vi "Unloading_OPEN_DOOR_ON_LOADED_status_Check.vi"(7 "CYCLE DATA IN":T1, 8 "error in":errorcluster) -> (0 "error out":errorcluster, 2 "search valid ?":bool, 5 "CYCLE DATA OUT":T1)   [LabVIEW 2017]
uses:
  Controls/Unload_Cyc_Data.ctl
  <vilib>/Utility/file.llb/Read Delimited Spreadsheet (string).vi
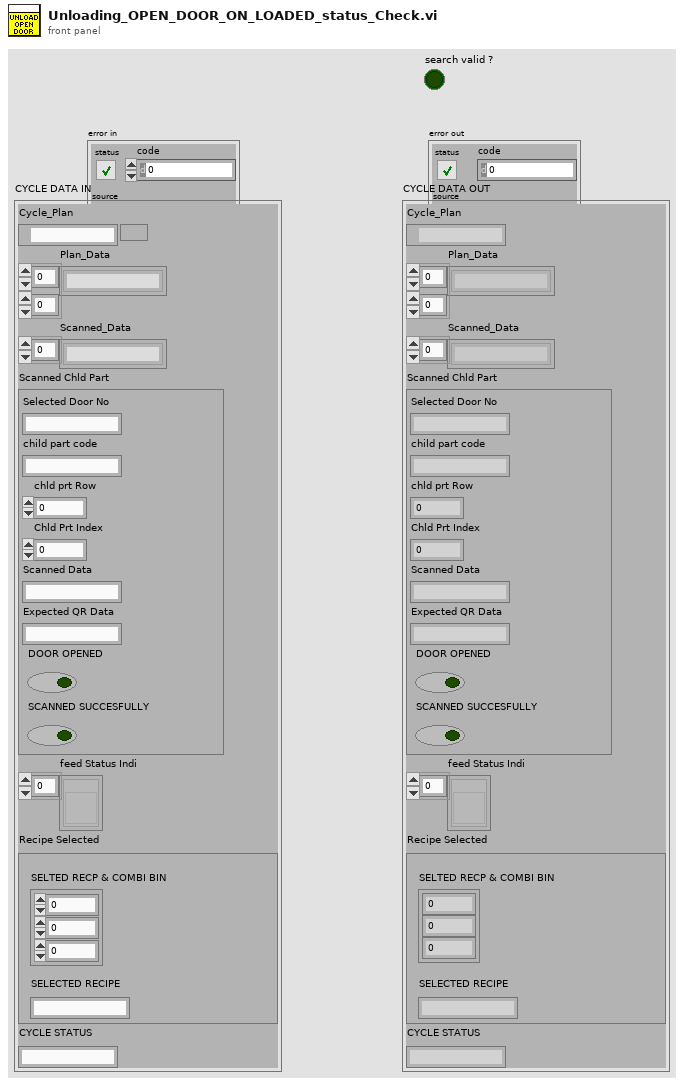
[diagram p1: front panel]
types:
  T1 = typedef "Unload_Cyc_Data.ctl" = cluster{"Cycle_Plan":path, "Plan_Data":string[][], "Scanned_Data":string[], "Scanned Chld Part":cluster{"Selected Door No":string, "child part code":string, "chld prt Row":i32, "Chld Prt Index":i32, "Scanned Data":string, "Expected QR Data":string, "DOOR OPENED":bool, "SCANNED SUCCESFULLY":bool}, "feed Status Indi":refnum<vi>[], "Recipe Selected":cluster{"SELTED RECP & COMBI BIN":cluster{"RECIPE INDEX":i32, "COMBI BIN":i32, "Section row no.":i32}, "SELECTED RECIPE":string}, "CYCLE STATUS":string}
  T2 = cluster{"RECIPE INDEX":i32, "COMBI BIN":i32, "Section row no.":i32}
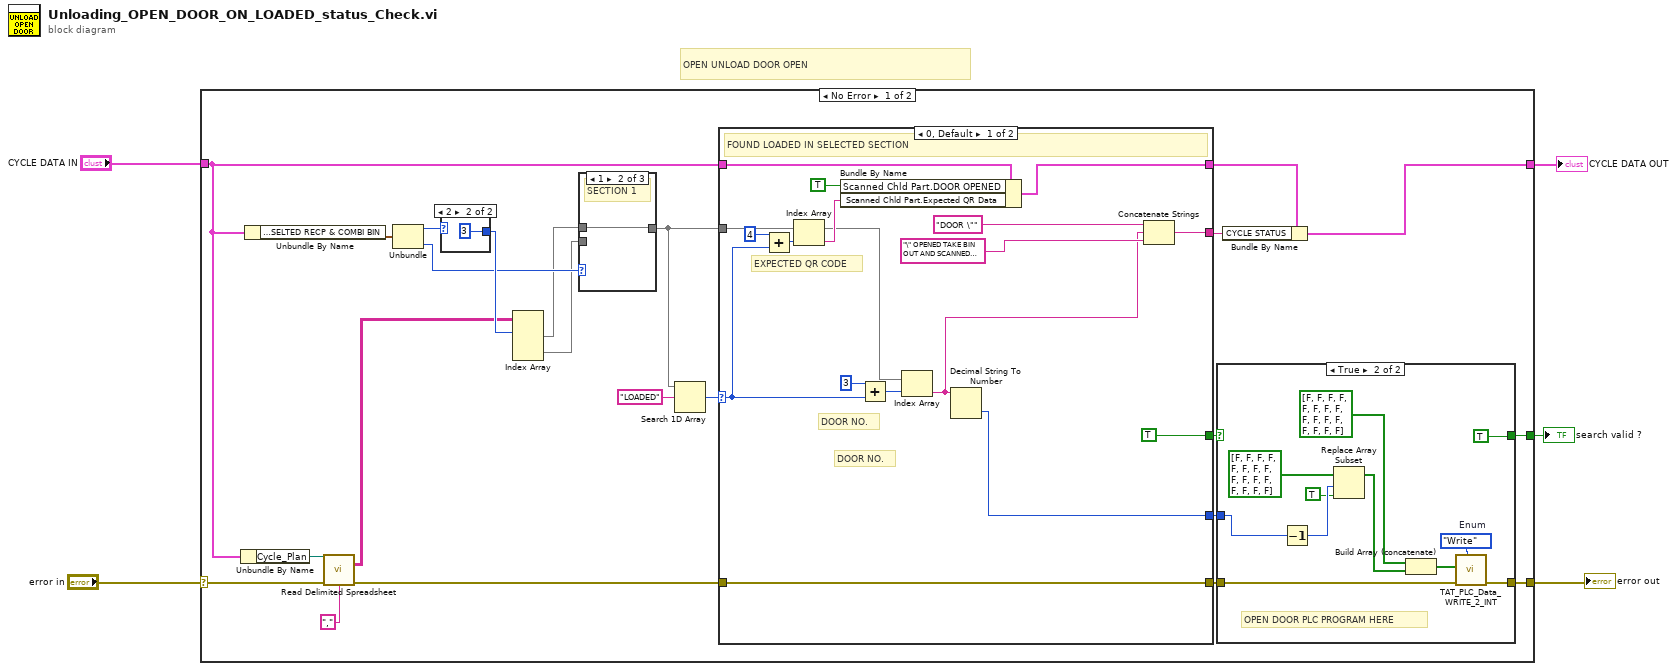
[diagram p0: block diagram]
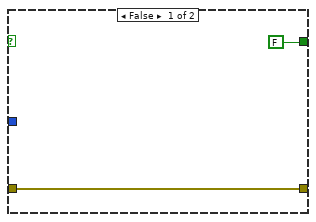
[diagram p2: hidden frame]
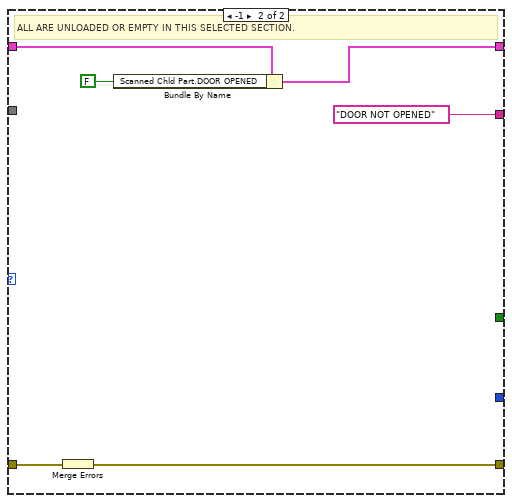
[diagram p3: hidden frame]
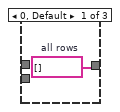
[diagram p4: hidden frame]
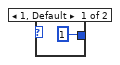
[diagram p6: hidden frame]
diagram:
  # "OPEN UNLOAD DOOR OPEN"
  n1 = case shown="No Error" "error in" {
    selector: "error in" -> [w25 w71]
    tunnel: [w18 w71] -> w4
    tunnel: [w13 w70] -> w2
    tunnel: "CYCLE DATA IN" -> [w21 w70]
    tunnel: [w15 _] -> w1
    frame No Error {
      n2 = Unbundle By Name(w21) -> ("Cycle_Plan"=w26:path)
      n3 = Unbundle By Name(w21) -> ("Recipe Selected.SELTED RECP & COMBI BIN"=w23:T2)
      n4 = call-poly <vilib>:"Read Delimited Spreadsheet.vi"("file path (dialog if empty)"=w26, "error in (no error)"=w25, "delimiter (\\t)"=",") -> ("all rows"=w19:string[][], "error out"=w24:errorcluster)  [unwired: 7 in, 4 out]
      n5 = Unbundle(w23) -> ("RECIPE INDEX"=w22:i32, "Section row no."=w11:i32)  [unwired: 1 out]
      n6 = case shown="2" w22 {
        tunnel: [1 3] -> w20
        frame 1, Default {
        }
        frame 2 {
        }
      }
      n7 = Index Array(array=w19, index (row) #1=w20) -> (element #1=w10:string[], element #2=w9:string[])  [unwired: 3 in]
      n8 = case shown="1" w11 {
        tunnel: w10 -> [_ w66 _]
        tunnel: w9 -> [_ _ w67]
        tunnel: [w65 w66 w67] -> w7
        frame 0, Default {
          w65 = string[] []  # all rows
        }
        frame 1 {
          # "SECTION 1"
        }
        frame 2 {
          # "SECTION 2"
        }
      }
      n9 = Search 1D Array(1D array=w7, element="LOADED") -> (index of element=w6:i32)  [unwired: 1 in]
      n10 = case shown="0, Default" w6 {
        selector: w6 -> [w48 _]
        tunnel: [w58 w63] -> w28
        tunnel: w24 -> [w58 w64]
        tunnel: [w55 w60] -> w14
        tunnel: w21 -> [w56 w61]
        tunnel: [TRUE _] -> w17
        tunnel: [w45 _] -> w16
        tunnel: [w44 "DOOR NOT OPENED"] -> w12
        tunnel: w7 -> [w52 _]
        frame 0, Default {
          # "DOOR NO."
          # "DOOR NO."
          # "EXPECTED QR CODE"
          # "FOUND LOADED IN SELECTED SECTION"
          n11 = Add(x=4, y=w48) -> (x+y=w47:i32)
          n12 = Index Array(array=w52, index=w47) -> (element=w54:string)
          n13 = Bundle By Name(cluster=w56, "Scanned Chld Part.DOOR OPENED"=TRUE, "Scanned Chld Part.Expected QR Data"=w54) -> (w55:T1)
          n14 = Add(x=3, y=w48) -> (x+y=w51:i32)
          n15 = Index Array(array=w52, index=w51) -> (element=w42:string)
          n16 = Decimal String To Number(string=w42) -> (number=w45:i32)  [unwired: 2 in, 1 out]
          n17 = Concatenate Strings("DOOR \"", w42, "\" OPENED TAKE BIN OUT AND SCANNED CODE.") -> (w44:string)
        }
        frame -1 {
          # "ALL ARE UNLOADED OR EMPTY IN THIS SELECTED SECTION."
          n18 = Merge Errors(w64) -> (w63:errorcluster)
          n19 = Bundle By Name(cluster=w61, "Scanned Chld Part.DOOR OPENED"=FALSE) -> (w60:T1)
        }
      }
      n20 = case shown="True" w17 {
        tunnel: w28 -> [w30 w37]
        tunnel: [w30 w36] -> w18
        tunnel: w16 -> [_ w31]
        tunnel: [FALSE TRUE] -> w15
        frame False {
        }
        frame True {
          w41 = enum16{"Read", "Write"}."Write"  # Enum
          # "OPEN DOOR PLC PROGRAM HERE"
          n21 = Decrement(x=w31) -> (x-1=w39:i32)
          n22 = Replace Array Subset(array=bool[] [FALSE, FALSE, FALSE, FALSE, FALSE, FALSE, FALSE, FALSE, FALSE, FALSE, FALSE, FALSE, FALSE, FALSE, FALSE, FALSE], new element=TRUE, index=w39) -> (w34:bool[])
          n23 = Build Array (concatenate)(bool[] [FALSE, FALSE, FALSE, FALSE, FALSE, FALSE, FALSE, FALSE, FALSE, FALSE, FALSE, FALSE, FALSE, FALSE, FALSE, FALSE], w34) -> (w35:bool[])
          n24 = call "TAT_PLC_Data_WRITE_2_INT.vi"("Enum"=w41, "error in (no error)"=w37, "Array"=w35) -> ("error out"=w36:errorcluster)  [unwired: 7 in, 1 out]
        }
      }
      n25 = Bundle By Name(cluster=w14, "CYCLE STATUS"=w12) -> (w13:T1)
    }
    frame Error {
    }
  }
  "error out" <- w4
  "CYCLE DATA OUT" <- w2
  "search valid ?" <- w1
